vi "ConfigOutputEnable.vi"(8 "error in (no error)":errorcluster, 11 "ClassIn":refnum<class "NiPxi6733.lvclass">) -> (0 "error out":errorcluster, 3 "ClassOut":refnum<class "NiPxi6733.lvclass">)   [LabVIEW 2014, in "FGenPlugins.lvlib" / "NiPxi6733.lvclass"]
uses:
  NiPxi6733.lvclass
  <vilib>/DAQmx/write.llb/DAQmx Write (Analog 1D Wfm NChan NSamp).vi
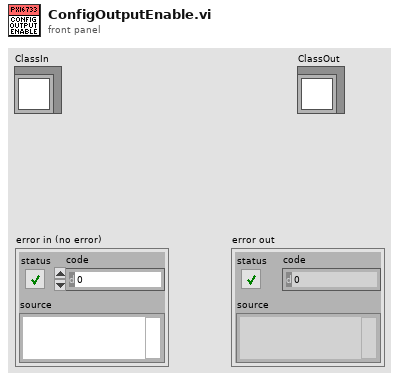
[diagram p1: front panel]
types:
  T1 = typedef "FGenPlugins.lvlib/NISTFGenPluginsBase.lvclass/ChannelParamElement.ctl" = cluster{"sName":string, "eOperateMode":u16, "bEnabled":bool, "eOutputMode":u16, "iIndex":i32, "iNameBufferSize":i32, "fGain":dbl}
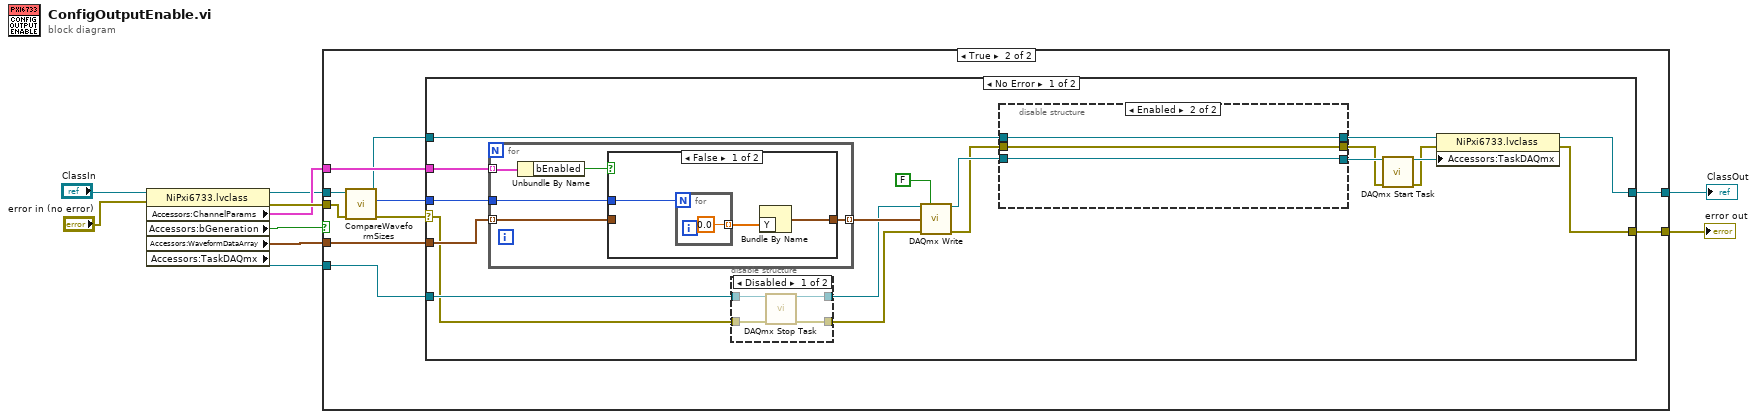
[diagram p0: block diagram]
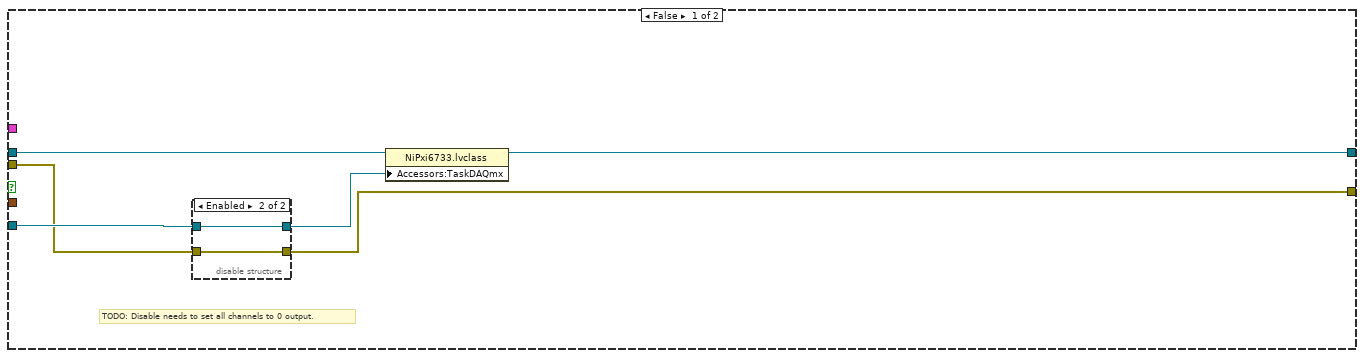
[diagram p2: hidden frame]
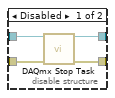
[diagram p3: hidden frame]
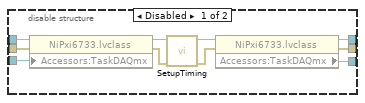
[diagram p5: hidden frame]
diagram:
  n1 = property class="NiPxi6733.lvclass"(reference="ClassIn") -> (reference out=w3:refnum<class "NiPxi6733.lvclass">, "Accessors:ChannelParams"=w4:T1[], "Accessors:bGeneration"=w5:bool, "Accessors:WaveformDataArray"=w2:waveform(dbl)[], "Accessors:TaskDAQmx"=w1:refnum<k21>)  [unwired: 1 in, 1 out]
  n2 = case shown="True" w5 {
    tunnel: w1 -> [w15 w27]
    tunnel: "error in (no error)" -> [w14 w30]
    tunnel: [w13 w28] -> w9
    tunnel: w4 -> [_ w31]
    tunnel: w2 -> [_ w25]
    tunnel: w3 -> [w12 w26]
    tunnel: [w11 w22] -> w8
    frame False {
      # "TODO: Disable needs to set all channels to 0 output."
      n3 = disable-structure shown="Enabled" {
        disable-tunnel: w15 -> [w19 w21]
        disable-tunnel: w14 -> [w18 w20]
        disable-tunnel: [w17 w20] -> w13
        disable-tunnel: [w16 w21] -> w10
        frame Disabled {
          n4 = call <vilib>:"DAQmx Stop Task.vi"("task/channels in"=w19, "error in"=w18) -> ("task out"=w16:refnum<k21>, "error out"=w17:errorcluster)  [unwired: 12 in]
        }
        frame Enabled {
        }
      }
      n5 = property class="NiPxi6733.lvclass"(reference=w12, "Accessors:TaskDAQmx"=w10) -> (reference out=w11:refnum<class "NiPxi6733.lvclass">)  [unwired: 1 in, 1 out]
    }
    frame True {
      n6 = call "CompareWaveformSizes.vi"("error in (no error)"=w30, "ClassIn"=w26) -> ("error out"=w24:errorcluster, "WaveformSize"=w29:i32, "ClassOut"=w23:refnum<class "NiPxi6733.lvclass">)  [unwired: 7 in]
      n7 = case shown="No Error" w24 {
        selector: w24 -> [w46 w81]
        tunnel: w31 -> [w45 _]
        tunnel: w29 -> [w50 _]
        tunnel: [w33 w81] -> w28
        tunnel: w27 -> [w48 _]
        tunnel: w25 -> [w47 _]
        tunnel: w23 -> [w42 w80]
        tunnel: [w38 w80] -> w22
        frame No Error {
          n8 = for {
            tunnel: w45 -> [w74] mode=indexing
            tunnel: w47 -> [w70] mode=indexing
            tunnel: [w72] -> w49 mode=indexing
            tunnel: w50 -> [w71]
            n9 = Unbundle By Name(w74) -> ("bEnabled"=w73:bool)
            n10 = case shown="False" w73 {
              tunnel: w70 -> [_ w79]
              tunnel: [w75 w79] -> w72
              tunnel: w71 -> [w77 _]
              frame False {
                n11 = for {
                  N: w77 -> [_]
                  tunnel: [0.0] -> w76 mode=indexing
                }
                n12 = Bundle By Name("Y"=w76) -> (w75:waveform(dbl))  [unwired: 1 in]
              }
              frame True {
              }
            }
          }
          n13 = disable-structure shown="Disabled" {
            disable-tunnel: w48 -> [w54 w56]
            disable-tunnel: w46 -> [w53 w55]
            disable-tunnel: [w52 w56] -> w44
            disable-tunnel: [w51 w55] -> w43
            frame Disabled {
              n14 = call <vilib>:"DAQmx Stop Task.vi"("task/channels in"=w54, "error in"=w53) -> ("task out"=w52:refnum<k21>, "error out"=w51:errorcluster)  [unwired: 12 in]
            }
            frame Enabled {
            }
          }
          n15 = call-poly <vilib>:"DAQmx Write.vi"("task/channels in"=w44, "auto start"=FALSE, "data"=w49, "error in"=w43) -> ("task out"=w41:refnum<k21>, "error out"=w36:errorcluster)  [unwired: 9 in, 1 out]
          n16 = disable-structure shown="Enabled" {
            disable-tunnel: w42 -> [w66 w69]
            disable-tunnel: w41 -> [w63 w67]
            disable-tunnel: [w62 w69] -> w40
            disable-tunnel: [w61 w67] -> w39
            disable-tunnel: w36 -> [w60 w68]
            disable-tunnel: [w57 w68] -> w35
            frame Disabled {
              n17 = property class="NiPxi6733.lvclass"(reference=w66, error in=w60, "Accessors:TaskDAQmx"=w63) -> (reference out=w64:refnum<class "NiPxi6733.lvclass">, error out=w59:errorcluster)
              n18 = call "SetupTiming.vi"("error in (no error)"=w59, "ClassIn"=w64) -> ("error out"=w58:errorcluster, "ClassOut"=w65:refnum<class "NiPxi6733.lvclass">)  [unwired: 8 in]
              n19 = property class="NiPxi6733.lvclass"(reference=w65, error in=w58) -> (reference out=w62:refnum<class "NiPxi6733.lvclass">, error out=w57:errorcluster, "Accessors:TaskDAQmx"=w61:refnum<k21>)
            }
            frame Enabled {
            }
          }
          n20 = call <vilib>:"DAQmx Start Task.vi"("task/channels in"=w39, "error in"=w35) -> ("task out"=w37:refnum<k21>, "error out"=w34:errorcluster)  [unwired: 12 in]
          n21 = property class="NiPxi6733.lvclass"(reference=w40, error in=w34, "Accessors:TaskDAQmx"=w37) -> (reference out=w38:refnum<class "NiPxi6733.lvclass">, error out=w33:errorcluster)
        }
        frame Error {
        }
      }
    }
  }
  "error out" <- w9
  "ClassOut" <- w8
